vi "Startup Wizard.vi"() -> (0 "analysis?":string, 2 "Settings":T1={"Name of test"="ScratchPad", "Date"=timestamp(0 s since 1904-01-01), "Location"="Home", "Template"="ScratchPad", "Soundcard"="OCTA-CAPTURE", "resolution"=32, "Sampling rate"=48000, "Ch1 Gain "=10.0, "Ch2 Gain"=20.0, "Sample time (s)"=0.3, "Pre-trigger (s)"=0.001, "Hammer Threshold"=0.01, "Positions"=12, "Taps/Position"=5, "Set Names"="H,V", "Freq resolution"=1.0, "Hammer cutoff"=0.025, "Mic cutoff"=0.25, "Double bounce "=0.01, "Hammer Cal"=1.0, "dB Offset"=0.0, "Accel Cal"=1.0, "Vibrometer Cal"=1.0, "Mic Cal"=49.38, "Output"=2, "Voltage Cal"=13.8, "Vibrometer Port"="ASRL27::INSTR", "Range"=50, "High Pass"=2, "Bandwidth"=25, "X Range"=[{"Minimum"=200.0, "Maximum"=10000.0, "Increment"=2500.0, "Minor Increment"=500.0, "Start"=2500.0}, {"Minimum"=0.0, "Maximum"=0.05, "Increment"=0.025, "Minor Increment"=0.0025, "Start"=0.0}, {"Minimum"=0.0, "Maximum"=0.3, "Increment"=0.1, "Minor Increment"=0.01, "Start"=0.0}, {"Minimum"=200.0, "Maximum"=10000.0, "Increment"=10.0, "Minor Increment"=100.0, "Start"=1000.0}], "Y Range"=[{"Minimum"=-25.0, "Maximum"=0.0, "Increment"=5.0, "Minor Increment"=1.0, "Start"=-25.0}, {"Minimum"=-0.1, "Maximum"=0.1, "Increment"=0.05, "Minor Increment"=0.01, "Start"=-0.1}, {"Minimum"=-0.1, "Maximum"=0.1, "Increment"=0.05, "Minor Increment"=0.01, "Start"=-0.1}, {"Minimum"=-30.0, "Maximum"=30.0, "Increment"=5.0, "Minor Increment"=1.0, "Start"=-30.0}], "dB Spread"=40.0, "Trigger"=0, "Ch_1"=1, "Ch_2"=2, "flip?"=FALSE, "60Hz"=FALSE, "Time offset"=0.0, "Piezo Cal"=1.0, "Default Notes"=""} {"Ch_2" min=1 step=1; "Ch_1" min=1 max=100 step=1; "Trigger" items=["Hammer (force)", "Self-tap", "Spacebar"]; "Bandwidth" items=["1 kHz"=1, "5 kHz"=5, "10 kHz"=10, "25 kHz"=25, "50 kHz"=50, "100 kHz"=100]; "High Pass" items=["Off", "13 Hz", "104 Hz"]; "Range" items=["10 mm/s"=1, "20 mm/s"=2, "50 mm/s"=5, "100 mm/s"=10, "200 mm/s"=20, "500 mm/s"=50, "1 m/s"=100, "2 m/s"=200]; "Output" items=["Accelerometer", "Speed (from acceleration)", "Microphone", "Vibrometer", "Piezo"]; "Voltage Cal" format="%#_13g"; "Ch2 Gain" format="%#_13g"; "Ch1 Gain" format="%#_13g"; "Double bounce" min=0.0; "Mic cutoff" min=0.0 format="%#_4g"; "Hammer cutoff" min=0.0 format="%#_4g"; "Freq resolution" min=0.0; "Pre-trigger (s)" format="%#_13g"; "Date" format="%<%H:%M\n%d/%m/%y>T"; "resolution" items=["16 bit"=16, "24 bit"=24, "32 bit"=32]; "Sampling rate" items=["22050 samp/s"=22050, "44100 samp/s"=44100, "48000 samp/s"=48000]})   [LabVIEW 2022 SP3]
uses:
  PreferencesControl.ctl
  <vilib>/Utility/error.llb/Trim Whitespace One-Sided.vi
  Mic/Mic_Global.vi
panel:
  in  "Stop 2":bool
  in  "Stop":bool
  in  "Back":bool
  in  "Next":bool
  out "Tabs":T2(tab)
  in  "acquire":bool
  in  "view":bool
  in  "device:":u16(ring) items=["Built-in Microph", "Jump Desktop Audio", "ZoomAudioD"]
  in  "Hammer Port":u16(ring)=2 items=["Port 1"=1, "Port 2"=2]
  in  "Microphone Port":u16(ring)=1 items=["Port 1"=1, "Port 2"=2]
  in  "flip?":bool
  in  "Ch1 Gain":dbl=30.0 format="%#_13g"
  in  "Ch2 Gain":dbl=20.0 format="%#_13g"
  in  "Instrument Name":string="First Test"
  in  "sets":u16(ring) items=["Just Horizontal Plane", "Just Vertical Plane", "First Horizontal then Vertical"]
  in  "Positions":i16=12
  in  "Taps":i16=5
  in  "Instrument Notes":string
  # "Welcome to the Obie App"
  # "Instructions at http://sites.google.com/view/oberlinacoustics"
  # "Typical Test Structure"
  # "for measuring the effect of bridge placement on a Strad copy"
  # "Instrument\n  (Name)"
  # "Strad Copy 77"
  # "Bridge 1"
  # "Bridge 2"
  # "Bridge 3"
  # "Test\n (bridge location)"
  # "Set\n (orientation)"
  # "Horizonal"
  # "Vertical"
  # "Position\n (Hammer location)"
  # "Position 1"
  # "Position 2"
  # "Position 3"
  # "Tap\n (trial)"
  # "Tap 1"
  # "Tap 2"
  # "Tap 3"
  # "Each tap is saved as a raw data file, the FRF is computed and averaged for each position, then averaged across positions, then averaged across sets so that you can compare tests (in this case the effect of bridge placement)"
  # "Hz"
  # "dB"
  # "dB"
  # "sec"
  # "sec"
  # "mV/Pa"
  # "mV/m/s2"
  # "mV/mm/s"
  # "V/N"
  # "sec"
  # "sec"
  # "mV/N"
  # "a.u."
  # "a.u."
  # "sec"
  # "I want to..."
  # "Searching for tests"
  # "The Search button will let you search your tests.  Hit View Data below to load a sample dataset.   All spectral data are saved as real averages (AvR) or complex averages (AvC) across runs.  H stands for a horizontal set and V stands for a vertical set (see image to the right).  For more information on these methods, click on the oberlinacoustics link above.\n\nTry changing axis ranges, adding bands, changing line colors, and hit the Intrepret button for fun.  In the future, use Search or Browse to load your instrument data.\n\nHints:\n1. Zoom axis: double click on the min or max value on the x axis and type the desired number\n2. To share data, zoom into subsections of the plot, separate plots, etc, shift-click on any graph\n3. Bands - select some of the default ones or make your own (Edit) and export to Excel"
  # "Select your sound card"
  # "If your microphone is not in the list, check to make sure it is on and connected to the compter.  If not, connect and restart the software"
  # "Select your connection ports"
  # "Make sure these are connected correctly"
  # "Enter the gains on the sound card for each channel"
  # "Just double-click on the number and type the new one"
  # "Note: If you are not using the OctaCapture, just enter 0"
  # "Name your instrument"
  # "This is the parent folder that will contain all your tests on the instrument.  The test name will autogenerate."
  # "How many sets?"
  # "A set defines a number of mic positions grouped together.  For instance, we often group all the mic positions with the hammer tapping the bridge in the horizontal plane into one set (H) and all the ones in the vertical plane in another (V)"
  # "How many mic positions?"
  # "We typically use 12 different angle locations in each set"
  # "How many taps per position?"
  # "This is the number of hammer taps that will be averaged to give you a single FRF for each position"
  # "Add any notes about the test"
  # "Delete anything you do not want"
  # "Many more settings..."
  # "We will assume default settings for everything else.  In the future, if you use the New Test button you can either pick from an existing template, enter your own settings or enter and then save the settings as your own template.\n\nIn the future, I would recommend calibrating your microphone as well.\n\nNow to take some data - hit the Take Data button and then start swinging the hammer to initiate acquisition.  It should automatically detect the hammer hit and show you data."
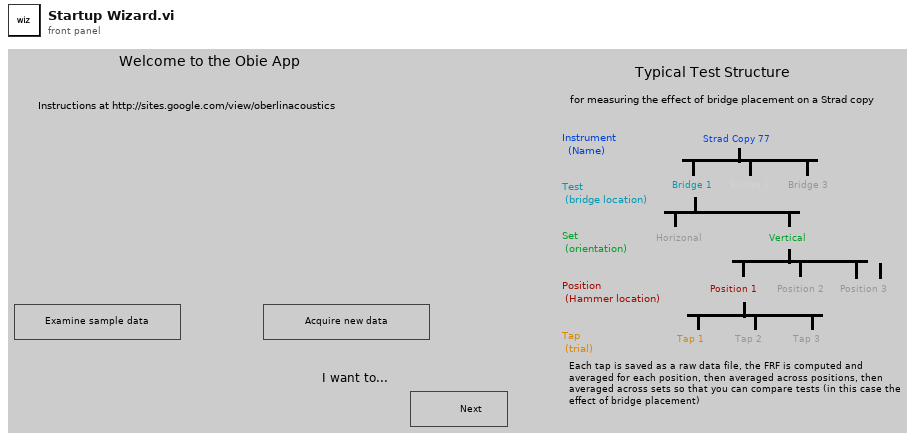
[diagram p1: front panel]
types:
  T1 = typedef "PreferencesControl.ctl" = cluster{"Name of test":string, "Date":timestamp, "Location":string, "Template":string, "Soundcard":string, "resolution":u16, "Sampling rate":u16, "Ch1 Gain ":dbl, "Ch2 Gain":dbl, "Sample time (s)":dbl, "Pre-trigger (s)":dbl, "Hammer Threshold":dbl, "Positions":i16, "Taps/Position":i16, "Set Names":string, "Freq resolution":dbl, "Hammer cutoff":dbl, "Mic cutoff":dbl, "Double bounce ":dbl, "Hammer Cal":dbl, "dB Offset":dbl, "Accel Cal":dbl, "Vibrometer Cal":dbl, "Mic Cal":dbl, "Output":u16, "Voltage Cal":dbl, "Vibrometer Port":refnum<visa-resource-name>, "Range":u16, "High Pass":u16, "Bandwidth":u16, "X Range":cluster{"Minimum":dbl, "Maximum":dbl, "Increment":dbl, "Minor Increment":dbl, "Start":dbl}[], "Y Range":cluster{"Minimum":dbl, "Maximum":dbl, "Increment":dbl, "Minor Increment":dbl, "Start":dbl}[], "dB Spread":dbl, "Trigger":u16, "Ch_1":u8, "Ch_2":u8, "flip?":bool, "60Hz":bool, "Time offset":dbl, "Piezo Cal":dbl, "Default Notes":string}
  T2 = enum32{"a or a", "plots", "get mic", "Ports", "Gains", "name", "sets", "positions", "taps", "Notes", "Done"}
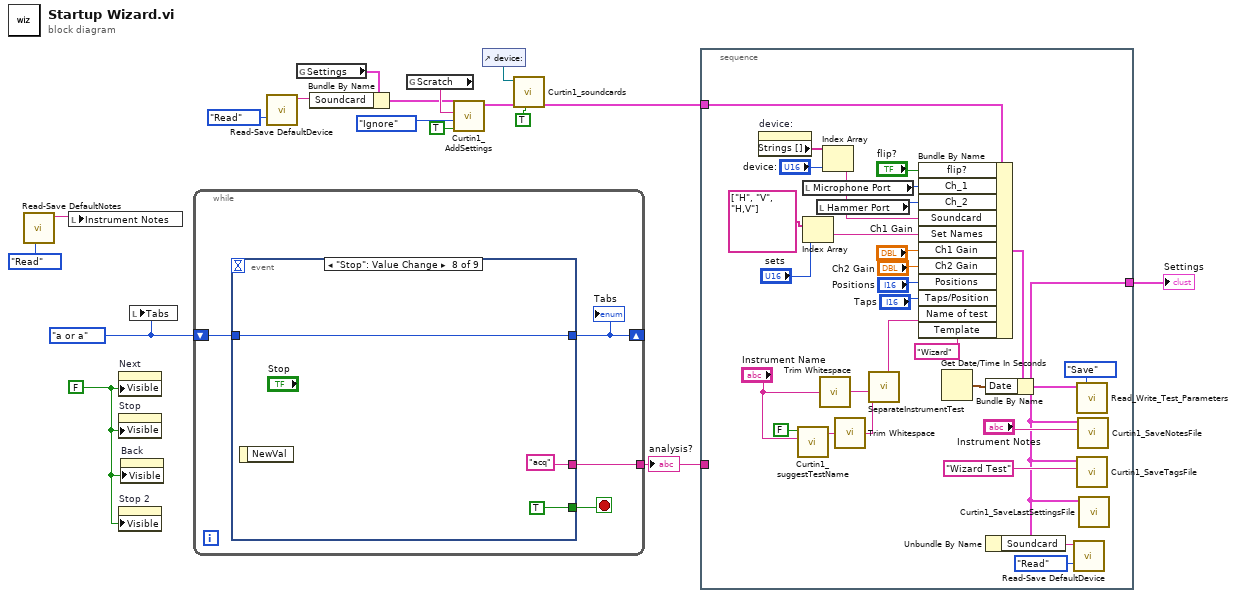
[diagram p0: block diagram]
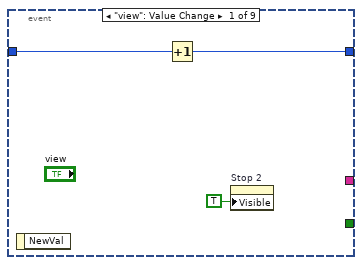
[diagram p2: hidden frame]
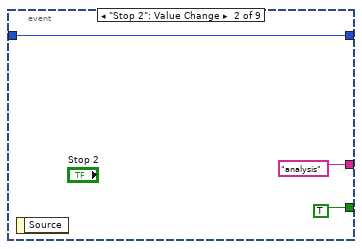
[diagram p3: hidden frame]
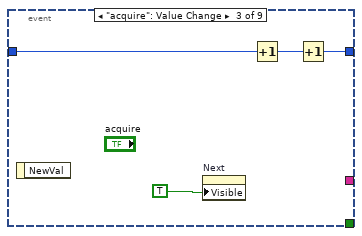
[diagram p4: hidden frame]
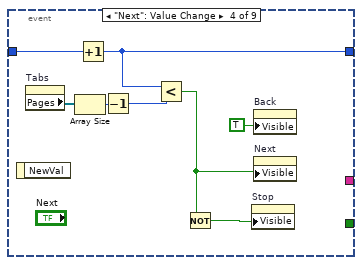
[diagram p5: hidden frame]
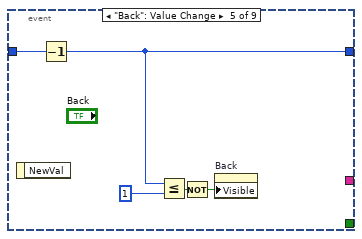
[diagram p6: hidden frame]
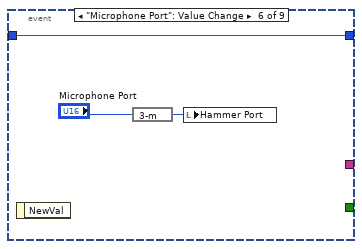
[diagram p7: hidden frame]
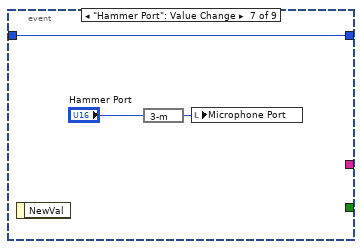
[diagram p8: hidden frame]
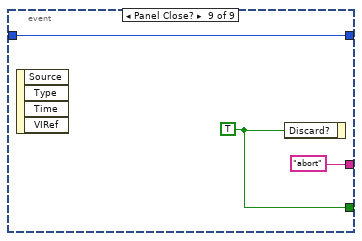
[diagram p9: hidden frame]
diagram:
  w10 = T2."a or a" ("Tabs")
  w14 = FALSE ("Visible")
  n1 = call "Read-Save DefaultNotes.vi"("Task"=enum16{"Save", "Read"}."Read") -> ("Notes Out"=w15:string)  [unwired: 9 in, 1 out]
  n2 = local write "Instrument Notes"(w15) -> ()
  n3 = property on="Next" class="Bool"("Visible"=w14) -> ()  [unwired: 2 in, 2 out]
  n4 = property on="Stop" class="Bool"("Visible"=w14) -> ()  [unwired: 2 in, 2 out]
  n5 = property on="Stop 2" class="Bool"("Visible"=w14) -> ()  [unwired: 2 in, 2 out]
  n6 = property on="Back" class="Bool"("Visible"=w14) -> ()  [unwired: 2 in, 2 out]
  n7 = local write "Tabs"(w10) -> ()
  n8 = while {
    shift-right: [w18] -> _
    shift-left: w10 -> [w20]
    tunnel: [w19] -> w1
    stop <- w21 stop-if-true
    n9 = event shown="[7] \"Stop\": Value Change" {
      selector: _ -> [_ _ _ _ _ _ _ _ _]
      dyn-events: _ -> [_ _ _ _ _ _ _ _ _]
      timeout: _ -> [_ _ _ _ _ _ _ _ _]
      tunnel: [_ TRUE ("Discard?") _ _ _ _ _ TRUE ("Discard?") w54] -> w21
      tunnel: [w23 w25 w30 w33 w41 w47 w50 w53 w56] -> w18
      tunnel: w20 -> [w24 w25 w31 w34 w44 w47 w50 w53 w56]
      tunnel: [_ "analysis" _ _ _ _ _ "acq" "abort"] -> w19
      event "view": Value Change {
        n10 = event-data() -> ()  [unwired: 1 in, 1 out]
        n11 = Increment(x=w24) -> (x+1=w23:T2)
        n12 = property on="Stop 2" class="Bool"("Visible"=TRUE) -> ()  [unwired: 2 in, 2 out]
      }
      event "Stop 2": Value Change {
        n13 = event-data() -> ()  [unwired: 1 in, 1 out]
      }
      event "acquire": Value Change {
        n14 = event-data() -> ()  [unwired: 1 in, 1 out]
        n15 = property on="Next" class="Bool"("Visible"=TRUE) -> ()  [unwired: 2 in, 2 out]
        n16 = Increment(x=w31) -> (x+1=w28:T2)
        n17 = Increment(x=w28) -> (x+1=w30:T2)
      }
      event "Next": Value Change {
        n18 = event-data() -> ()  [unwired: 1 in, 1 out]
        n19 = property on="Tabs" class="TabCtl (strict)"() -> ("Pages"=w38:refnum<vi>[])  [unwired: 2 in, 2 out]
        n20 = Array Size(array=w38) -> (size(s)=w37:i32)
        n21 = Increment(x=w34) -> (x+1=w33:T2)
        n22 = Decrement(x=w37) -> (x-1=w32:i32)
        n23 = Less?(x=w33, y=w32) -> (x < y?=w36:bool)
        n24 = Not(x=w36) -> (.not. x?=w39:bool)
        n25 = property on="Stop" class="Bool"("Visible"=w39) -> ()  [unwired: 2 in, 2 out]
        n26 = property on="Back" class="Bool"("Visible"=TRUE) -> ()  [unwired: 2 in, 2 out]
        n27 = property on="Next" class="Bool"("Visible"=w36) -> ()  [unwired: 2 in, 2 out]
      }
      event "Back": Value Change {
        n28 = event-data() -> ()  [unwired: 1 in, 1 out]
        n29 = Decrement(x=w44) -> (x-1=w41:T2)
        n30 = Less Or Equal?(x=w41, y=1) -> (x <= y?=w42:bool)
        n31 = Not(x=w42) -> (.not. x?=w40:bool)
        n32 = property on="Back" class="Bool"("Visible"=w40) -> ()  [unwired: 2 in, 2 out]
      }
      event "Microphone Port": Value Change {
        n33 = event-data() -> ()  [unwired: 1 in, 1 out]
        n34 = expression code="3-m"("Microphone Port") -> (w45:u16)
        n35 = local write "Hammer Port"(w45) -> ()
      }
      event "Hammer Port": Value Change {
        n36 = event-data() -> ()  [unwired: 1 in, 1 out]
        n37 = expression code="3-m"("Hammer Port") -> (w48:u16)
        n38 = local write "Microphone Port"(w48) -> ()
      }
      event "Stop": Value Change {
        n39 = event-data() -> ()  [unwired: 1 in, 1 out]
      }
      event Panel Close? {
        w54 = TRUE ("Discard?")
        n40 = event-data() -> ()  [unwired: 1 in, 4 out]
        n41 = event-data("Discard?"=w54) -> ()  [unwired: 1 in, 1 out]
      }
    }
    "Tabs" <- w18
  }
  "analysis?" <- w1
  n42 = call "Read-Save DefaultDevice.vi"("Task"=enum16{"Save", "Read"}."Read") -> ("Soundcard Out"=w8:string)  [unwired: 9 in, 1 out]
  n43 = global read "Mic_Global.vi" "Settings"() -> (w7:T1)
  n44 = Bundle By Name(cluster=w7, "Soundcard"=w8) -> (w3:T1)
  n45 = global read "Mic_Global.vi" "Scratch"() -> (w5:string)
  n46 = call "Curtin1_AddSettings.vi"("Date?"=TRUE, "Check?"=enum16{"Ignore", "Check", "Replace"}."Ignore", "Template"=w5, "Settings in"=w3) -> ("Settings Out"=w2:T1)  [unwired: 6 in, 1 out]
  n47 = control-ref of="device:"() -> (w13:refnum<vi>)
  n48 = call "Curtin1_soundcards.vi"("hush?"=TRUE, "Settings In"=w2, "device:"=w13) -> ("Settings Out"=w11:T1)  [unwired: 7 in, 1 out]
  n49 = stacked-sequence {
    tunnel: [w60] -> w17
    tunnel: w11 -> [w58]
    tunnel: w1 -> [_]
    frame #0 {
      n50 = property on="device:" class="Ring (strict)"() -> ("Strings []"=w70:string[])  [unwired: 2 in, 2 out]
      n51 = call "Curtin1_suggestTestName.vi"("instrument"="Instrument Name", "Build?"=FALSE) -> ("Suggested Test"=w72:string)  [unwired: 9 in]
      n52 = local read "Microphone Port"() -> (w64:u16)
      n53 = Index Array(array=string[] ["H", "V", "H,V"], index="sets") -> (element=w66:string)
      n54 = local read "Hammer Port"() -> (w65:u16)
      n55 = call <vilib>:"Trim Whitespace.vi"("string"="Instrument Name") -> ("trimmed string"=w76:string)  [unwired: 1 in]
      n56 = Index Array(array=w70, index="device:") -> (element=w69:string)
      n57 = call <vilib>:"Trim Whitespace.vi"("string"=w72) -> ("trimmed string"=w75:string)  [unwired: 1 in]
      n58 = call "SeparateInstrumentTest.vi"("test in"=w75, "Instrument in"=w76) -> ("Instrument -- test out"=w71:string)  [unwired: 5 in, 4 out]
      n59 = Bundle By Name(cluster=w58, "flip?"="flip?", "Ch_1"=w64, "Ch_2"=w65, "Soundcard"=w69, "Set Names"=w66, "Ch1 Gain"="Ch1 Gain", "Ch2 Gain"="Ch2 Gain", "Positions"="Positions", "Taps/Position"="Taps", "Name of test"=w71, "Template"="Wizard") -> (w78:T1)
      n60 = Get Date/Time In Seconds() -> (seconds since 1Jan1904=w81:timestamp)
      n61 = Bundle By Name(cluster=w78, "Date"=w81) -> (w60:T1)
      n62 = Unbundle By Name(w60) -> ("Soundcard"=w59:string)
      n63 = call "Read-Save DefaultDevice.vi"("Task"=enum16{"Save", "Read"}."Read", "Soundcard"=w59) -> ()  [unwired: 8 in, 2 out]
      n64 = call "Read_Write_Test_Parameters.vi"("Task"=enum16{"Save", "Read", "Clear"}."Save", "Settings"=w60) -> ()  [unwired: 8 in, 2 out]
      n65 = call "Curtin1_SaveTagsFile.vi"("Tags"="Wizard Test", "Settings in"=w60) -> ()  [unwired: 10 in]
      n66 = call "Curtin1_SaveNotesFile.vi"("Notes"="Instrument Notes", "Settings in"=w60) -> ()  [unwired: 10 in]
      n67 = call "Curtin1_SaveLastSettingsFile.vi"("Settings in"=w60) -> ()  [unwired: 11 in]
    }
  }
  "Settings" <- w17
